vi "GetDBAL_class.vi"(8 "error in (no error)":errorcluster, 11 "FAMM in":refnum<class "FAMM.lvclass">) -> (0 "error out":errorcluster, 2 "DBAL_class":refnum<data-value>, 3 "FAMM out":refnum<class "FAMM.lvclass">)   [LabVIEW 2014, in "FAMM.lvclass"]
doc: "Read database Class"
uses:
  FAMM.lvclass
  DBAL/DBAL.lvclass
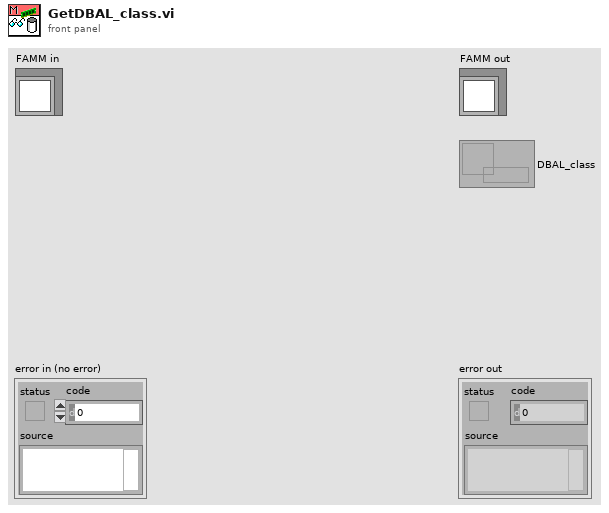
[diagram p1: front panel]
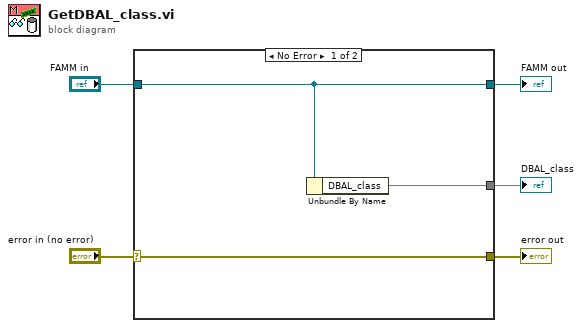
[diagram p0: block diagram]
diagram:
  n1 = case shown="No Error" "error in (no error)" {
    selector: "error in (no error)" -> [w7 w9]
    tunnel: [w7 w9] -> w4
    tunnel: [w6 w10] -> w2
    tunnel: "FAMM in" -> [w6 w10]
    tunnel: [w8 _] -> w1
    frame No Error {
      n2 = Unbundle By Name(w6) -> ("DBAL_class"=w8)
    }
    frame Error {
    }
  }
  "error out" <- w4
  "FAMM out" <- w2
  "DBAL_class" <- w1
